vi "AppConfig.vi"(8 "error in (no error)":errorcluster, 11 "RingdownPlugin":refnum<class "RingdownPlugin.lvclass">=refnum) -> (0 "error out":errorcluster, 3 "RingdownPlugin out":refnum<class "RingdownPlugin.lvclass">)   [LabVIEW 2017, in "AppPlugins.lvlib" / "RingdownPlugin.lvclass"]
uses:
  RingdownPlugin.lvclass
  PronyConfig.ctl
  PublicAPI/TypeDef/RingdownConfig.ctl
  PublicAPI/TypeDef/ePhase.ctl
  RingdownPlugin.lvclass/RingdownPlugin.ctl
  Accessors/Read RingdownConfig.vi
  Accessors/Write RingdownConfig.vi
panel:
  in  "Phase":T1 items=["A", "B", "C"]
  in  "WinSize":u32 caption="Window Size"
  in  "EndOffset":u32 caption="Final Offset (ms)" max=0
  in  "StOffset":i32 caption="Start Offset (ms)" min=0
  out "RingdownConfig":T2={"Config"={"Addmod"=-1, "Scalmod"=0, "Lpocon"=-1, "Pircon"=-1, "Dmodes"=0, "Lpmcon"=3, "Lpacon"=3, "Fbcon"=1, "Ordcon"=1, "Trimre"=-1.0, "Ftrimh"=-1.0, "Ftriml"=-1.0}, "Window"={"StOffset"=0, "EndOffset"=0, "Length"=0}, "V index"=0, "I index"=3, "PosSeq"=FALSE} {"Config"."Fbcon" items=["", "Forward", "Forward-Backward", "Backward"]; "Config"."Lpmcon" items=["", "Correlation", "Pre-windowed", "Covariance", "Post-windowed"]; "Config"."Lpacon" items=["", "SVD with possible rank reduction", "QR reduction via LAPACK", "Total least squares via SVD"]}
  in  "Cancel Button":bool
  in  "Save Button":bool
  in  "Prony Configuration":T3={"Lpmcon"=3, "Lpacon"=3, "Fbcon"=1, "LPOrd"={"Auto"=TRUE, "Val"=116}, "UTrimFreq"={"Auto"=TRUE, "Val"=20.0}, "LTrimFreq"={"Auto"=TRUE, "Val"=0.0}, "ResTrim"={"Auto"=TRUE, "Val"=1e-08}} {"Fbcon" items=["", "Forward", "Forward-Backward", "Backward"]; "Lpacon" items=["", "SVD with possible rank reduction", "QR reduction via LAPACK", "Total least squares via SVD"]; "Lpmcon" items=["", "Correlation", "Pre-windowed", "Covariance", "Post-windowed"]}
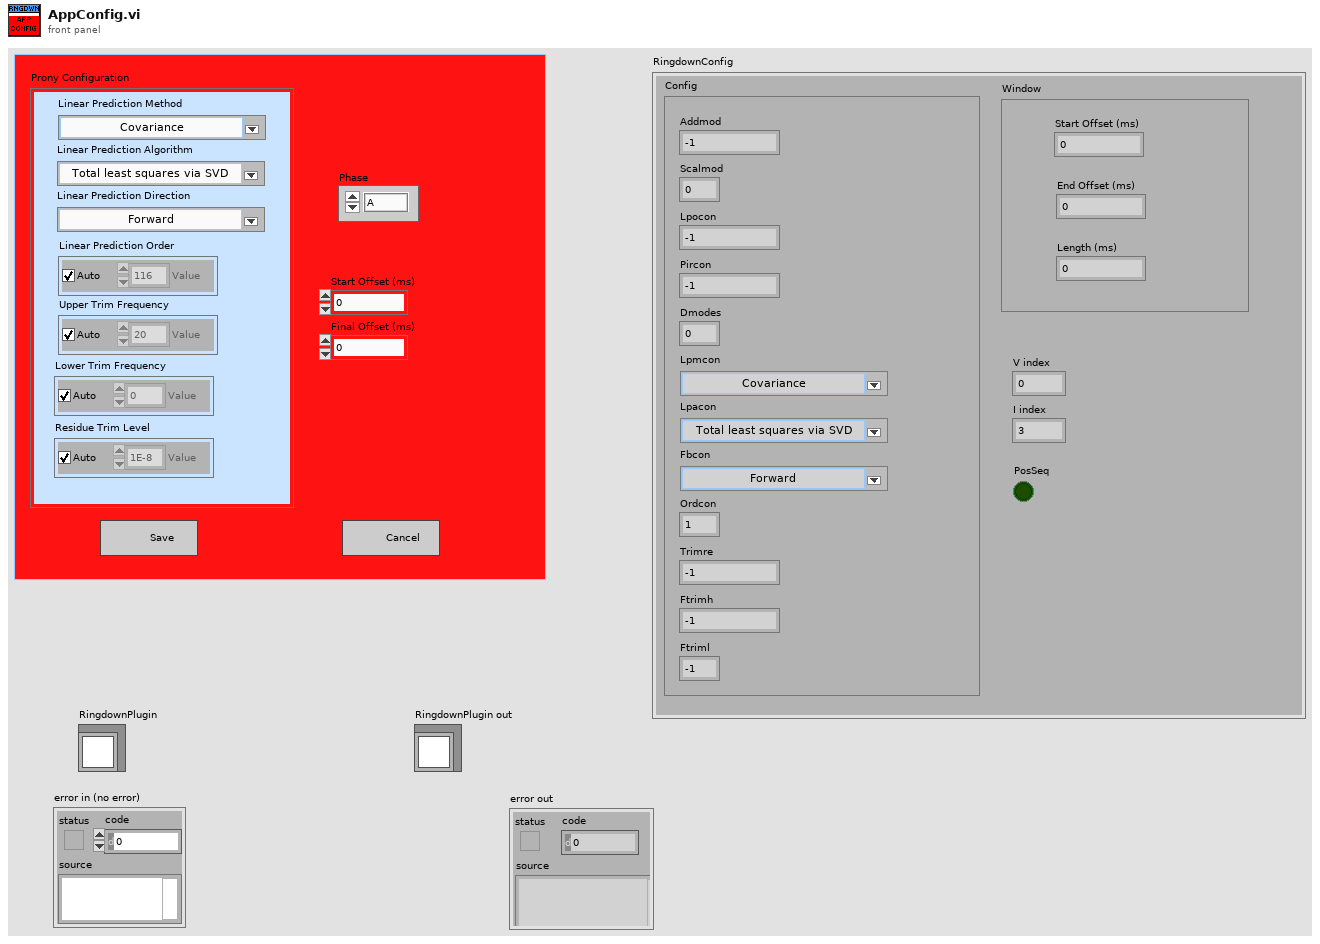
[diagram p1: front panel]
types:
  T1 = typedef "AppPlugins.lvlib/RingdownPlugin.lvclass/ePhase.ctl" = u16
  T2 = typedef "AppPlugins.lvlib/RingdownPlugin.lvclass/RingdownConfig.ctl" = cluster{"Config":cluster{"Addmod":i32, "Scalmod":i32, "Lpocon":i32, "Pircon":i32, "Dmodes":i32, "Lpmcon":u16, "Lpacon":u16, "Fbcon":u16, "Ordcon":i32, "Trimre":dbl, "Ftrimh":dbl, "Ftriml":dbl}, "Window":cluster{"StOffset":i32, "EndOffset":i32, "Length":i32}, "V index":i32, "I index":i32, "PosSeq":bool}
  T3 = typedef "AppPlugins.lvlib/RingdownPlugin.lvclass/PronyConfig.ctl" = cluster{"Lpmcon":u16, "Lpacon":u16, "Fbcon":u16, "LPOrd":cluster{"Auto":bool, "Val":i32}, "UTrimFreq":cluster{"Auto":bool, "Val":dbl}, "LTrimFreq":cluster{"Auto":bool, "Val":dbl}, "ResTrim":cluster{"Auto":bool, "Val":dbl}}
  T4 = enum8{"Enabled", "Disabled", "Disabled and Grayed Out"}
  T5 = typedef "PronyConfig.ctl" = cluster{"Lpmcon":u16, "Lpacon":u16, "Fbcon":u16, "LPOrd":cluster{"Auto":bool, "Val":i32}, "UTrimFreq":cluster{"Auto":bool, "Val":dbl}, "LTrimFreq":cluster{"Auto":bool, "Val":dbl}, "ResTrim":cluster{"Auto":bool, "Val":dbl}}
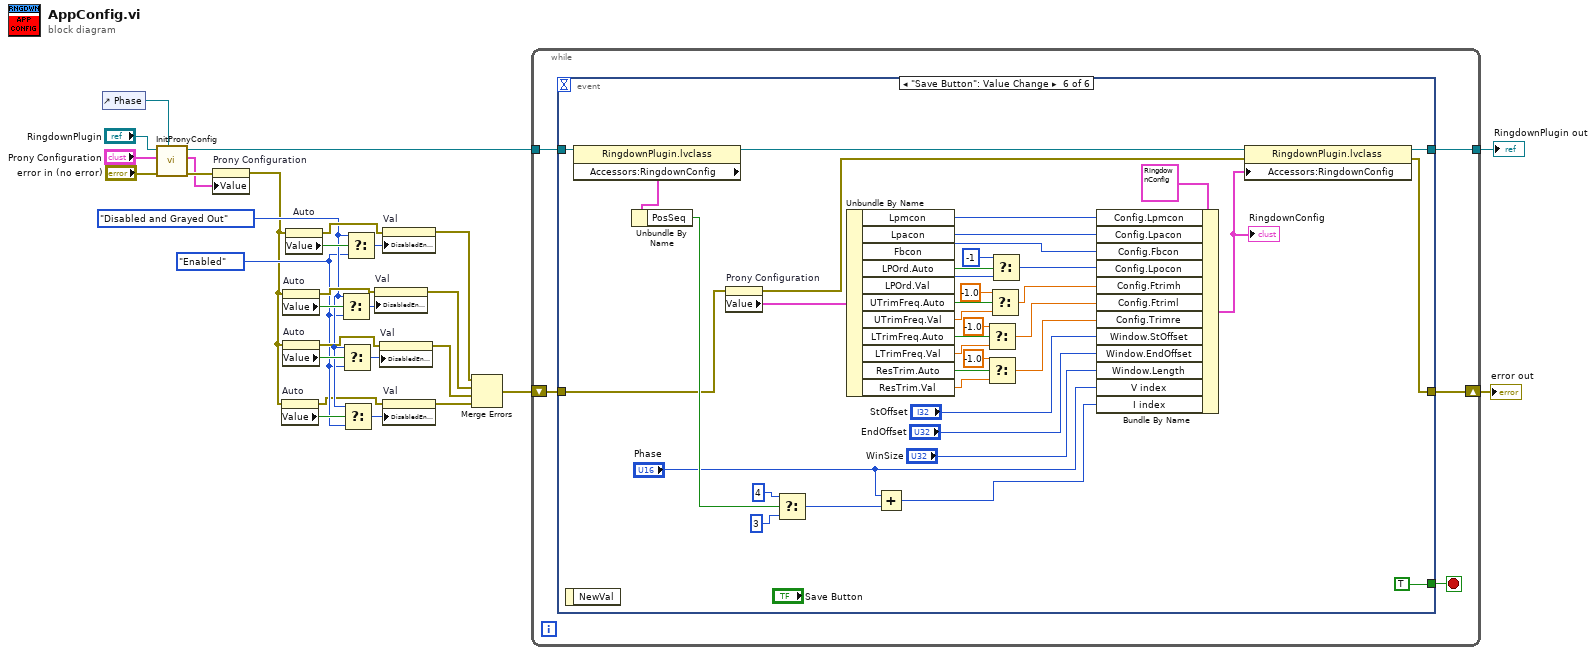
[diagram p0: block diagram]
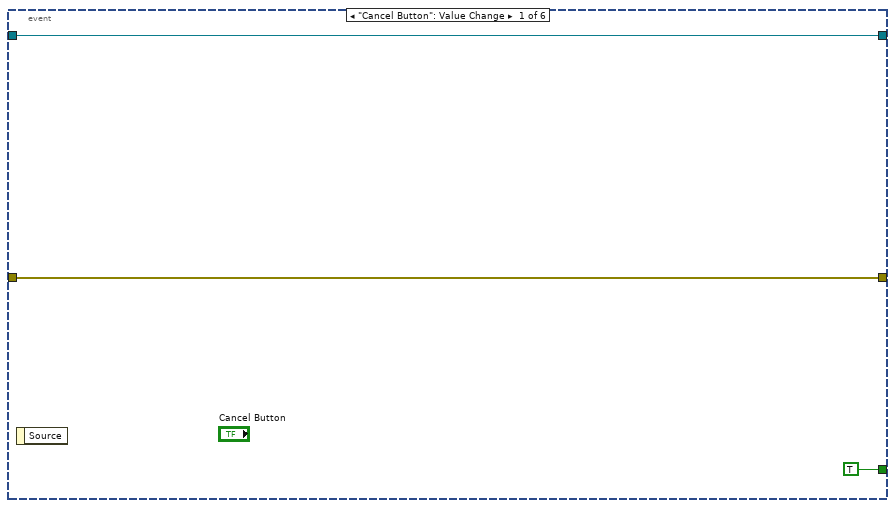
[diagram p2: hidden frame]
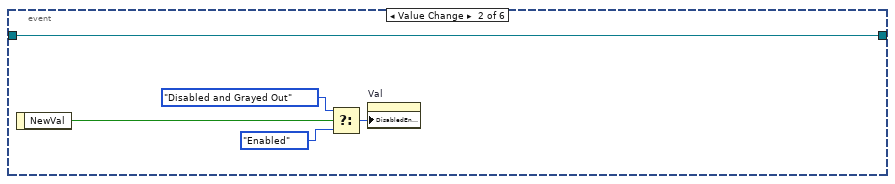
[diagram p3: hidden frame]
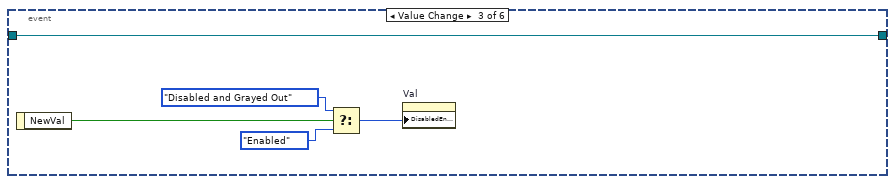
[diagram p4: hidden frame]
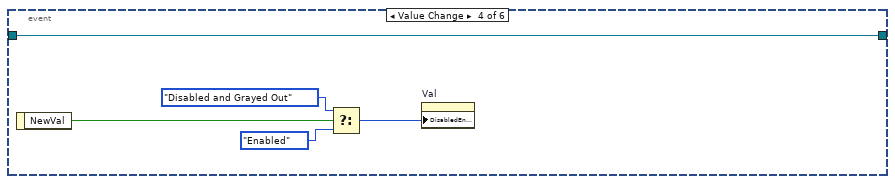
[diagram p5: hidden frame]
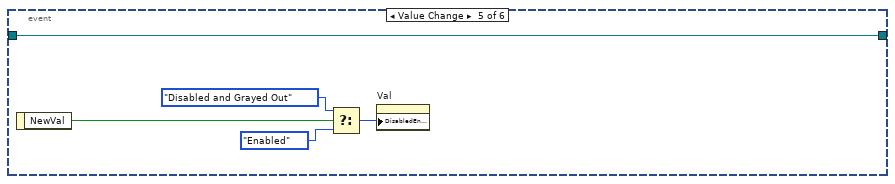
[diagram p6: hidden frame]
diagram:
  w13 = T4."Disabled and Grayed Out" ("Disabled")
  w12 = T4."Enabled" ("Disabled")
  n1 = control-ref of="Phase"() -> (w1:refnum<vi>)
  n2 = call "InitPronyConfig.vi"("Ring Refnum"=w1, "error in (no error)"="error in (no error)", "Prony Configuration"="Prony Configuration", "RingdownPlugin"="RingdownPlugin") -> ("error out"=w4:errorcluster, "Prony Configuration"=w2:T3, "RingdownPlugin"=w26:refnum<class "RingdownPlugin.lvclass">)  [unwired: 5 in]
  n3 = property on="Prony Configuration" class="Clust (strict)"(error in=w4, "Value"=w2) -> (error out=w3:errorcluster)  [unwired: 1 in, 1 out]
  n4 = property on="Auto" class="Bool (strict)"(error in=w3) -> (error out=w10:errorcluster, "Value"=w14:bool)  [unwired: 1 in, 1 out]
  n5 = property on="Auto" class="Bool (strict)"(error in=w3) -> (error out=w18:errorcluster, "Value"=w20:bool)  [unwired: 1 in, 1 out]
  n6 = property on="Auto" class="Bool (strict)"(error in=w3) -> (error out=w15:errorcluster, "Value"=w17:bool)  [unwired: 1 in, 1 out]
  n7 = property on="Auto" class="Bool (strict)"(error in=w3) -> (error out=w21:errorcluster, "Value"=w23:bool)  [unwired: 1 in, 1 out]
  n8 = Select(t=w13, s=w20, f=w12) -> (s? t:f=w19:T4)
  n9 = Select(t=w13, s=w17, f=w12) -> (s? t:f=w16:T4)
  n10 = Select(t=w13, s=w14, f=w12) -> (s? t:f=w11:T4)
  n11 = Select(t=w13, s=w23, f=w12) -> (s? t:f=w22:T4)
  n12 = property on="Val" class="DigNum (strict)"(error in=w18, "DisabledEnum"=w19) -> (error out=w8:errorcluster)  [unwired: 1 in, 1 out]
  n13 = property on="Val" class="DigNum (strict)"(error in=w15, "DisabledEnum"=w16) -> (error out=w7:errorcluster)  [unwired: 1 in, 1 out]
  n14 = property on="Val" class="DigNum (strict)"(error in=w21, "DisabledEnum"=w22) -> (error out=w9:errorcluster)  [unwired: 1 in, 1 out]
  n15 = property on="Val" class="DigNum (strict)"(error in=w10, "DisabledEnum"=w11) -> (error out=w6:errorcluster)  [unwired: 1 in, 1 out]
  n16 = Merge Errors(w9, w8, w7, w6) -> (w5:errorcluster)
  n17 = while {
    shift-right: [w34] -> w29
    shift-left: w5 -> [w31]
    tunnel: w26 -> [w32]
    tunnel: [w33] -> w28
    stop <- w30 stop-if-true
    n18 = event shown="[5] \"Save Button\": Value Change" {
      selector: _ -> [_ _ _ _ _ _]
      dyn-events: _ -> [_ _ _ _ _ _]
      timeout: _ -> [_ _ _ _ _ _]
      tunnel: [w36 _ _ _ _ w96] -> w34
      tunnel: [w37 w38 w43 w48 w53 w95] -> w33
      tunnel: w32 -> [w37 w38 w43 w48 w53 w94]
      tunnel: w31 -> [w36 _ _ _ _ w59]
      tunnel: [TRUE _ _ _ _ TRUE] -> w30
      event "Cancel Button": Value Change {
        n19 = event-data() -> ()  [unwired: 1 in, 1 out]
      }
      event Value Change {
        n20 = event-data() -> ("NewVal"=w42:bool)  [unwired: 1 in]
        n21 = Select(t=T4."Disabled and Grayed Out" ("Disabled"), s=w42, f=T4."Enabled" ("Disabled")) -> (s? t:f=w39:T4)
        n22 = property on="Val" class="DigNum (strict)"("DisabledEnum"=w39) -> ()  [unwired: 2 in, 2 out]
      }
      event Value Change {
        n23 = event-data() -> ("NewVal"=w47:bool)  [unwired: 1 in]
        n24 = Select(t=T4."Disabled and Grayed Out" ("Disabled"), s=w47, f=T4."Enabled" ("Disabled")) -> (s? t:f=w44:T4)
        n25 = property on="Val" class="DigNum (strict)"("DisabledEnum"=w44) -> ()  [unwired: 2 in, 2 out]
      }
      event Value Change {
        n26 = event-data() -> ("NewVal"=w52:bool)  [unwired: 1 in]
        n27 = Select(t=T4."Disabled and Grayed Out" ("Disabled"), s=w52, f=T4."Enabled" ("Disabled")) -> (s? t:f=w49:T4)
        n28 = property on="Val" class="DigNum (strict)"("DisabledEnum"=w49) -> ()  [unwired: 2 in, 2 out]
      }
      event Value Change {
        n29 = event-data() -> ("NewVal"=w57:bool)  [unwired: 1 in]
        n30 = Select(t=T4."Disabled and Grayed Out" ("Disabled"), s=w57, f=T4."Enabled" ("Disabled")) -> (s? t:f=w54:T4)
        n31 = property on="Val" class="DigNum (strict)"("DisabledEnum"=w54) -> ()  [unwired: 2 in, 2 out]
      }
      event "Save Button": Value Change {
        n32 = event-data() -> ()  [unwired: 1 in, 1 out]
        n33 = property class="RingdownPlugin.lvclass"(reference=w94) -> (reference out=w65:refnum<class "RingdownPlugin.lvclass">, "Accessors:RingdownConfig"=w64:T2)  [unwired: 1 in, 1 out]
        n34 = Unbundle By Name(w64) -> ("PosSeq"=w63:bool)
        n35 = property on="Prony Configuration" class="Clust (strict)"(error in=w59) -> (error out=w71:errorcluster, "Value"=w72:T5)  [unwired: 1 in, 1 out]
        n36 = Select(t=u16 4 ("y"), s=w63, f=u16 3 ("y")) -> (s? t:f=w60:u16)
        n37 = Unbundle By Name(w72) -> ("Lpmcon"=w90:u16, "Lpacon"=w88:u16, "Fbcon"=w87:u16, "LPOrd.Auto"=w93:bool, "LPOrd.Val"=w92:i32, "UTrimFreq.Auto"=w86:bool, "UTrimFreq.Val"=w85:dbl, "LTrimFreq.Auto"=w81:bool, "LTrimFreq.Val"=w80:dbl, "ResTrim.Auto"=w77:bool, "ResTrim.Val"=w76:dbl)
        n38 = Add(x="Phase", y=w60) -> (x+y=w66:T1)
        n39 = Select(t=-1.0, s=w81, f=w80) -> (s? t:f=w78:dbl)
        n40 = Select(t=-1.0, s=w77, f=w76) -> (s? t:f=w74:dbl)
        n41 = Select(t=-1.0, s=w86, f=w85) -> (s? t:f=w82:dbl)
        n42 = Select(t=-1, s=w93, f=w92) -> (s? t:f=w83:i32)
        n43 = Bundle By Name(cluster=T2 {"Config"={"Addmod"=-1, "Scalmod"=0, "Lpocon"=-1, "Pircon"=-1, "Dmodes"=0, "Lpmcon"=3, "Lpacon"=1, "Fbcon"=1, "Ordcon"=1, "Trimre"=-1.0, "Ftrimh"=-1.0, "Ftriml"=-1.0}, "Window"={"StOffset"=1, "EndOffset"=601, "Length"=10000}, "V index"=0, "I index"=1, "PosSeq"=FALSE} ("RingdownConfig"), "Config.Lpmcon"=w90, "Config.Lpacon"=w88, "Config.Fbcon"=w87, "Config.Lpocon"=w83, "Config.Ftrimh"=w82, "Config.Ftriml"=w78, "Config.Trimre"=w74, "Window.StOffset"="StOffset", "Window.EndOffset"="EndOffset", "Window.Length"="WinSize", "V index"="Phase", "I index"=w66) -> (w70:T2)
        "RingdownConfig" <- w70
        n44 = property class="RingdownPlugin.lvclass"(reference=w65, error in=w71, "Accessors:RingdownConfig"=w70) -> (reference out=w95:refnum<class "RingdownPlugin.lvclass">, error out=w96:errorcluster)
      }
    }
  }
  "error out" <- w29
  "RingdownPlugin out" <- w28
